vi "Write SensorInfo Changed Event.vi"(8 "error in (no error)":errorcluster, 10 "SensorInfo Changed Event":refnum<user-event>, 11 "SensorView in":refnum<class "SensorView.lvclass">) -> (0 "error out":errorcluster, 3 "SensorView out":refnum<class "SensorView.lvclass">)   [LabVIEW 2012, in "Sensor Definition.lvlib" / "SensorView.lvclass"]
uses:
  SensorView.lvclass
  SensorInfo.lvclass
  SensorView.lvclass/SensorView.ctl
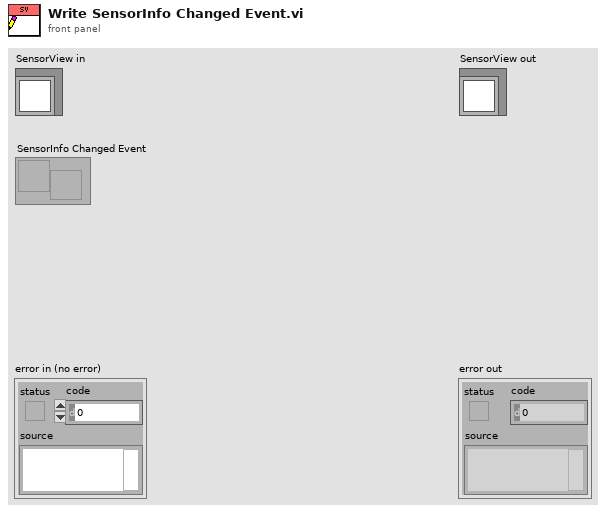
[diagram p1: front panel]
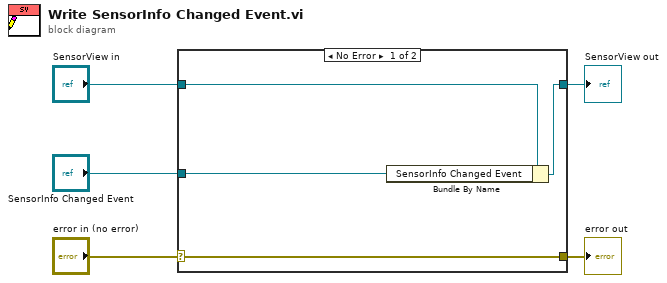
[diagram p0: block diagram]
diagram:
  n1 = case shown="No Error" "error in (no error)" {
    selector: "error in (no error)" -> [w9 w10]
    tunnel: [w9 w10] -> w4
    tunnel: [w7 w11] -> w2
    tunnel: "SensorView in" -> [w8 w11]
    tunnel: "SensorInfo Changed Event" -> [w6 _]
    frame No Error {
      n2 = Bundle By Name(cluster=w8, "SensorInfo Changed Event"=w6) -> (w7:refnum<class "SensorView.lvclass">)
    }
    frame Error {
    }
  }
  "error out" <- w4
  "SensorView out" <- w2
